vi "ConvertTo(AC d).vi"(8 "error in":errorcluster, 9 "Message Payload":variant) -> (0 "error out":errorcluster, 1 "Message Payload  waveform":waveform(dbl))   [LabVIEW 2017]
doc: "Convert variant to DAQmx waveform type\n\nBolder Software LLC"
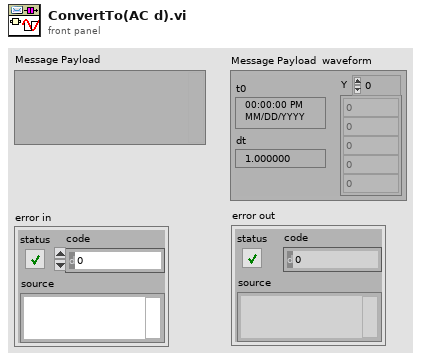
[diagram p1: front panel]
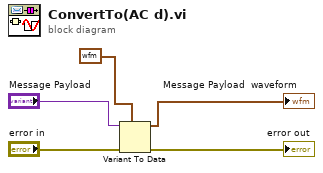
[diagram p0: block diagram]
diagram:
  n1 = Variant To Data(error in="error in", type=waveform(dbl) {"t0"=timestamp(0 s since 1904-01-01), "dt"=1.0, "Y"=[]} ("Message Payload  waveform"), Variant="Message Payload") -> (data=→"Message Payload  waveform":waveform(dbl), error out=→"error out":errorcluster)
